vi "pointA.vi"   [LabVIEW 2011]
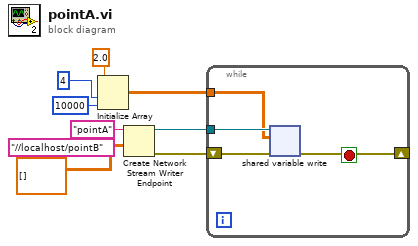
[diagram p0: block diagram]
diagram:
  n1 = Initialize Array(2.0 ("element"), 4 ("dimension size"), 10000 ("dimension size")) -> (w2:dbl[][])
  n2 = Create Network Stream Writer Endpoint(9:dbl[][] [], 10:"//localhost/pointB" ("reader url"), 11:"pointA" ("writer name")) -> (0:w8:errorcluster, 3:w9:refnum<k21>)  [unwired: 3 in]
  n3 = while {
    tunnel: w9 -> [w12]
    tunnel: w2 -> [w11]
    shift-right: [w10] -> _
    shift-left: w8 -> [w13]
    stop <- w10 stop-if-true
    n4 = shared-variable-write(w12, w13, w11) -> (w10:errorcluster)  [unwired: 1 in, 2 out]
  }
